vi "StringConverter.vi"(11 "Composer Command":string[](array[string])) -> (0 "Internal Channel Delay and Width":dbl[][](array[numeric]), 3 "Internal Channel Name":string[](array[string]), 8 "Mux Value":i32[](array[numeric]))   [LabVIEW 2012]
uses:
  <vilib>/regexp/Match Regular Expression.xnode
panel:
  out "Internal State":string[][](array[string])
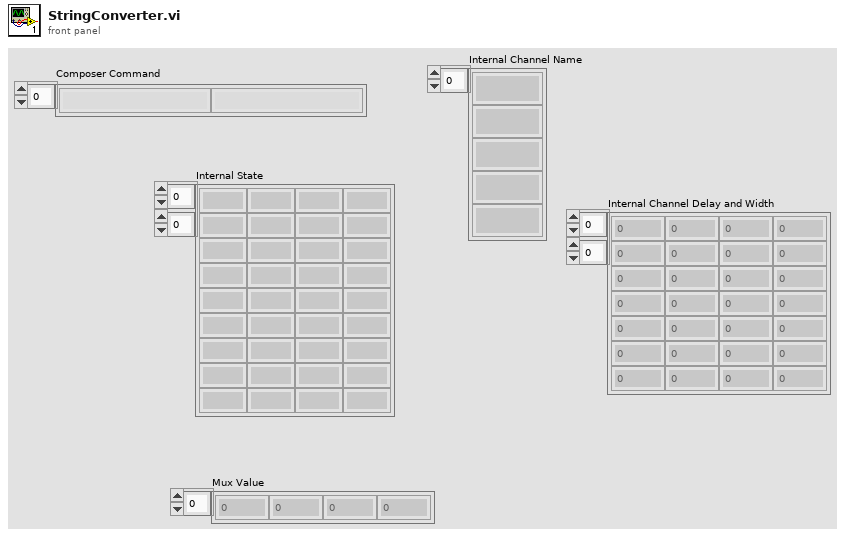
[diagram p1: front panel]
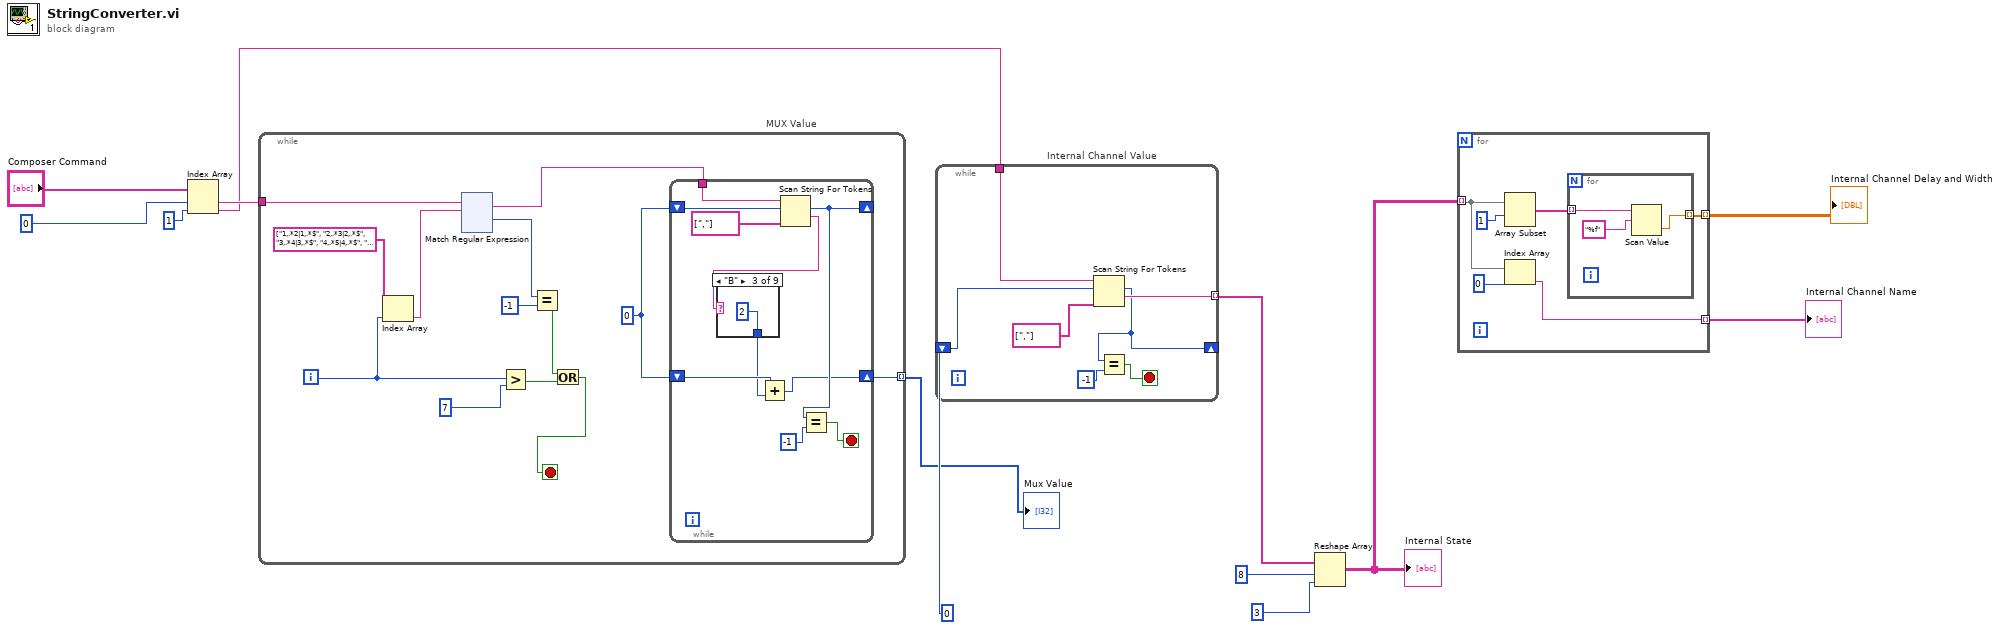
[diagram p0: block diagram]
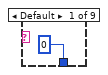
[diagram p2: hidden frame]
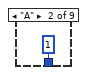
[diagram p3: hidden frame]
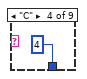
[diagram p4: hidden frame]
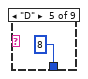
[diagram p5: hidden frame]
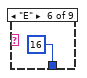
[diagram p6: hidden frame]
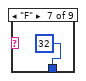
[diagram p7: hidden frame]
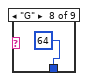
[diagram p8: hidden frame]
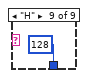
[diagram p9: hidden frame]
diagram:
  n1 = Index Array(array="Composer Command", index #1=0, index #2=1) -> (element #1=w5:string, element #2=w2:string)
  n2 = while "MUX Value" {
    tunnel: w5 -> [w14]
    tunnel: [w18] -> w1 mode=indexing
    i -> [w24]
    stop <- w20 stop-if-true
    w19 = 0
    n3 = Index Array(array=string[] ["1,.*2|1,.*$", "2,.*3|2,.*$", "3,.*4|3,.*$", "4,.*5|4,.*$", "5,.*6|5,.*$", "6,.*7|6,.*$", "7,.*8|7,.*$", "8,.*$"], index=w24) -> (element=w17:string)
    n4 = xnode "Match Regular Expression"("input string"=w14, "regular expression"=w17) -> ("whole match"=w16:string, "offset past match"=w15:i32)  [unwired: 4 in, 3 out]
    n5 = Greater?(x=w24, y=7) -> (0:w21:bool)
    n6 = Equal?(x=w15, y=-1) -> (x = y?=w22:bool)
    n7 = Or(x=w22, y=w21) -> (x .or. y?=w20:bool)
    n8 = while {
      tunnel: w16 -> [w146]
      shift-right: [w142] -> _
      shift-left: w19 -> [w143]
      shift-right: [w138] -> w18
      shift-left: w19 -> [w141]
      stop <- w144 stop-if-true
      n9 = Scan String For Tokens(6:string[] [","], 8:w143, 9:w146) -> (1:w140:string, 2:w142:i32)  [unwired: 3 in, 2 out]
      n10 = case shown="\"B\"" w140 {
        tunnel: [0 1 2 4 8 16 32 64 128] -> w139
        frame Default {
        }
        frame "A" {
        }
        frame "B" {
        }
        frame "C" {
        }
        frame "D" {
        }
        frame "E" {
        }
        frame "F" {
        }
        frame "G" {
        }
        frame "H" {
        }
      }
      n11 = Add(x=w141, y=w139) -> (x+y=w138:i32)
      n12 = Equal?(x=w142, y=-1) -> (x = y?=w144:bool)
    }
  }
  "Mux Value" <- w1
  n13 = while "Internal Channel Value" {
    shift-right: [w159] -> _
    shift-left: 0 -> [w158]
    tunnel: [w162] -> w12 mode=indexing
    tunnel: w2 -> [w157]
    stop <- w161 stop-if-true
    n14 = Scan String For Tokens(6:string[] [","], 8:w158, 9:w157) -> (1:w162:string, 2:w159:i32)  [unwired: 3 in, 2 out]
    n15 = Equal?(x=w159, y=-1) -> (x = y?=w161:bool)
  }
  n16 = Reshape Array(w12, 8, 3) -> (w9:string[][])
  "Internal State" <- w9
  n17 = for {
    tunnel: w9 -> [w166] mode=indexing
    tunnel: [w169] -> w8 mode=indexing
    tunnel: [w164] -> w7 mode=indexing
    n18 = Array Subset(array=w166, index=1) -> (w167:string[])  [unwired: 1 in]
    n19 = Index Array(array=w166, index=0) -> (element=w164:string)
    n20 = for {
      tunnel: w167 -> [w172] mode=indexing
      tunnel: [w170] -> w169 mode=indexing
      n21 = Scan Value(string=w172, format string="%f") -> (value=w170:dbl)  [unwired: 1 in, 1 out]
    }
  }
  "Internal Channel Delay and Width" <- w8
  "Internal Channel Name" <- w7
